vi "Ping All Dispatchers.vi"(5 "receiver port (0)":u16, 7 "ignore sender (T)":bool=TRUE, 9 "timeout (1000 ms)":i32=1000, 11 "error in":errorcluster) -> (4 "response messages":T1[](array[typedef]), 6 "response":string, 15 "error out":errorcluster)   [LabVIEW 2014, in "AMC.lvlib"]
doc: "Pings the Dispatchers in all applications that use \"receiver port\", then returns the replies received within the specified timeout.\n\nIf \"receiver port\" is undefined, this VI will attempt to use the default UDP port."
uses:
  AMC.lvlib
  Message.ctl
  <vilib>/NI/Tools/Keyed Array/KeyedArray.ctl
  <vilib>/NI/Tools/Keyed Array/Map String.vi
  <vilib>/NI/Tools/String/Get Case Matching.vi
  Globals.vi
  <vilib>/NI/Tools/Keyed Array/Tools_KeyedArray.lvlib
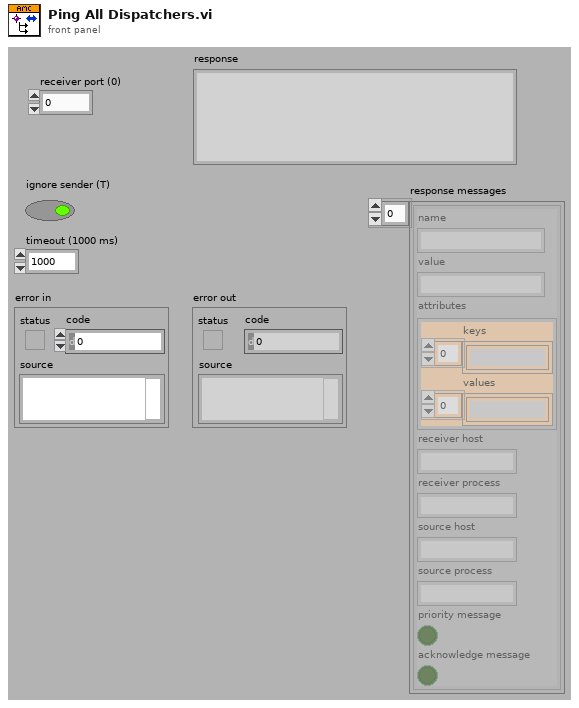
[diagram p1: front panel]
types:
  T1 = typedef "AMC.lvlib/Message.ctl" = cluster{"name":string, "value":string, "attributes":T2, "receiver host":string, "receiver process":string, "source host":string, "source process":string, "priority message":bool, "acknowledge message":bool}
  T2 = typedef "Tools_KeyedArray.lvlib/KeyedArray.ctl" = cluster{"keys":string[], "values":string[]}
  T3 = typedef "AMC.lvlib/Message Queue.ctl" = refnum<queue>
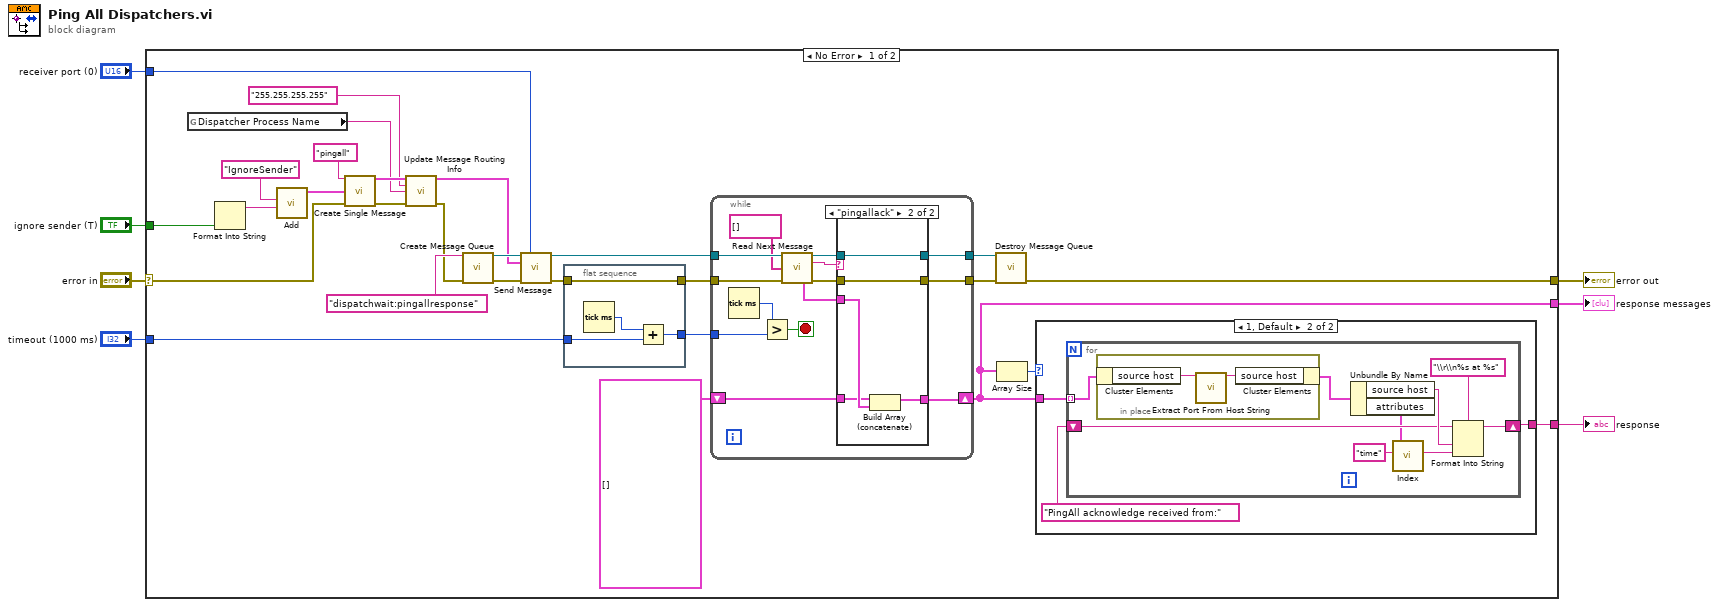
[diagram p0: block diagram]
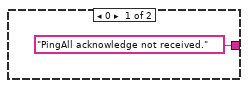
[diagram p2: hidden frame]
diagram:
  n1 = case shown="No Error" "error in" {
    selector: "error in" -> [w9 w77]
    tunnel: [w35 w77] -> w7
    tunnel: [w26 _] -> w6
    tunnel: [w25 _] -> w5
    tunnel: "ignore sender (T)" -> [w23 _]
    tunnel: "timeout (1000 ms)" -> [w20 _]
    tunnel: "receiver port (0)" -> [w8 _]
    frame No Error {
      n2 = global read "Globals.vi" "Dispatcher Process Name"() -> (w12:string)
      n3 = Format Into String(w23) -> (resulting string=w22:string)  [unwired: 3 in, 1 out]
      n4 = call <vilib>:"Add.vi"("value"=w22, "key"="IgnoreSender") -> ("array out"=w16:T2)  [unwired: 2 in, 3 out]
      n5 = call "Create Single Message.vi"("name"="pingall" ("Name"), "attributes"=w16, "error in"=w9) -> ("message"=w15:T1, "error out"=w11:errorcluster)  [unwired: 11 in]
      n6 = call "Update Message Routing Info.vi"("message"=w15, "receiver host (\"\")"="255.255.255.255" ("receiver host"), "receiver process (\"\")"=w12, "error in"=w11) -> ("message"=w14:T1, "error out"=w10:errorcluster)  [unwired: 10 in]
      n7 = call "Create Message Queue.vi"("message queue name"="dispatchwait:pingallresponse", "error in"=w10) -> ("message queue out"=w19:T3, "error out"=w29:errorcluster)  [unwired: 12 in]
      n8 = call "Send Message.vi"("message queue in"=w19, "receiver port"=w8, "message"=w14, "error in"=w29) -> ("message queue out"=w18:T3, "error out"=w34:errorcluster)  [unwired: 9 in, 1 out]
      n9 = flat-sequence {
        tunnel: [w54] -> w33
        tunnel: w34 -> [w54]
        tunnel: [w52] -> w32
        tunnel: w20 -> [w51]
        frame #0 {
          n10 = Tick Count (ms)() -> (millisecond timer value=w53:u32)
          n11 = Add(x=w53, y=w51) -> (x+y=w52:u32)
        }
      }
      n12 = while {
        tunnel: w33 -> [w68]
        tunnel: [w64] -> w30
        tunnel: [w63] -> w31
        tunnel: w18 -> [w62]
        tunnel: w32 -> [w60]
        shift-right: [w59] -> w25
        shift-left: T1[] [] -> [w58]
        stop <- w57 stop-if-true
        n13 = Tick Count (ms)() -> (millisecond timer value=w61:u32)
        n14 = Greater?(x=w61, y=w60) -> (0:w57:bool)
        n15 = call "Read Next Message.vi"("message queue in"=w62, "termination list ([Exit])"=string[] [], "error in"=w68) -> ("message queue out"=w65:T3, "message name"=w67:string, "message"=w56:T1, "error out"=w66:errorcluster)  [unwired: 5 in, 4 out]
        n16 = case shown="\"pingallack\"" w67 {
          tunnel: w56 -> [_ w73]
          tunnel: [w69 w74] -> w59
          tunnel: [w70 w76] -> w64
          tunnel: w66 -> [w70 w76]
          tunnel: [w71 w75] -> w63
          tunnel: w65 -> [w71 w75]
          tunnel: w58 -> [w69 w72]
          frame Default {
          }
          frame "pingallack" {
            n17 = Build Array (concatenate)(w72, w73) -> (w74:T1[])
          }
        }
      }
      n18 = call "Destroy Message Queue.vi"("message queue in"=w31, "error in"=w30) -> ("error out"=w35:errorcluster)  [unwired: 11 in, 2 out]
      n19 = Array Size(array=w25) -> (size(s)=w27:i32)
      n20 = case shown="1, Default" w27 {
        tunnel: ["PingAll acknowledge not received." w37] -> w26
        tunnel: w25 -> [_ w39]
        frame 0 {
        }
        frame 1, Default {
          n21 = for {
            shift-right: [w46] -> w37
            shift-left: "PingAll acknowledge received from:" ("format string") -> [w45]
            tunnel: w39 -> [w41] mode=indexing
            n22 = in-place {
              n23 = in-place-cluster #1(w41) -> ("source host"=w50:string)
              n24 = call "Extract Port From Host String.vi"("host in"=w50) -> ("host out"=w49:string)  [unwired: 12 in, 2 out]
              n25 = in-place-cluster #1("source host"=w49) -> (w40:T1)
            }
            n26 = Unbundle By Name(w40) -> ("source host"=w48:string, "attributes"=w43:T2)
            n27 = call <vilib>:"Index.vi"("key"="time", "array in"=w43) -> ("value"=w42:string)  [unwired: 2 in, 3 out]
            n28 = Format Into String(format string="\\r\\n%s at %s", initial string=w45, w48, w42) -> (resulting string=w46:string)  [unwired: 1 in, 1 out]
          }
        }
      }
    }
    frame Error {
    }
  }
  "error out" <- w7
  "response messages" <- w5
  "response" <- w6
